vi "Historical Warnings (SubVI).vi"(7 "Warnings bool array":bool[](array[boolean]), 8 "in":bool, 11 "warnings table in":T1(array[cluster]) {"Time Stamp" format="%<%.3X %x>T"}) -> (3 "Warnings table out":T1(array[cluster]) {"Time Stamp" format="%<%.3X %x>T"})   [LabVIEW 2022 SP3]
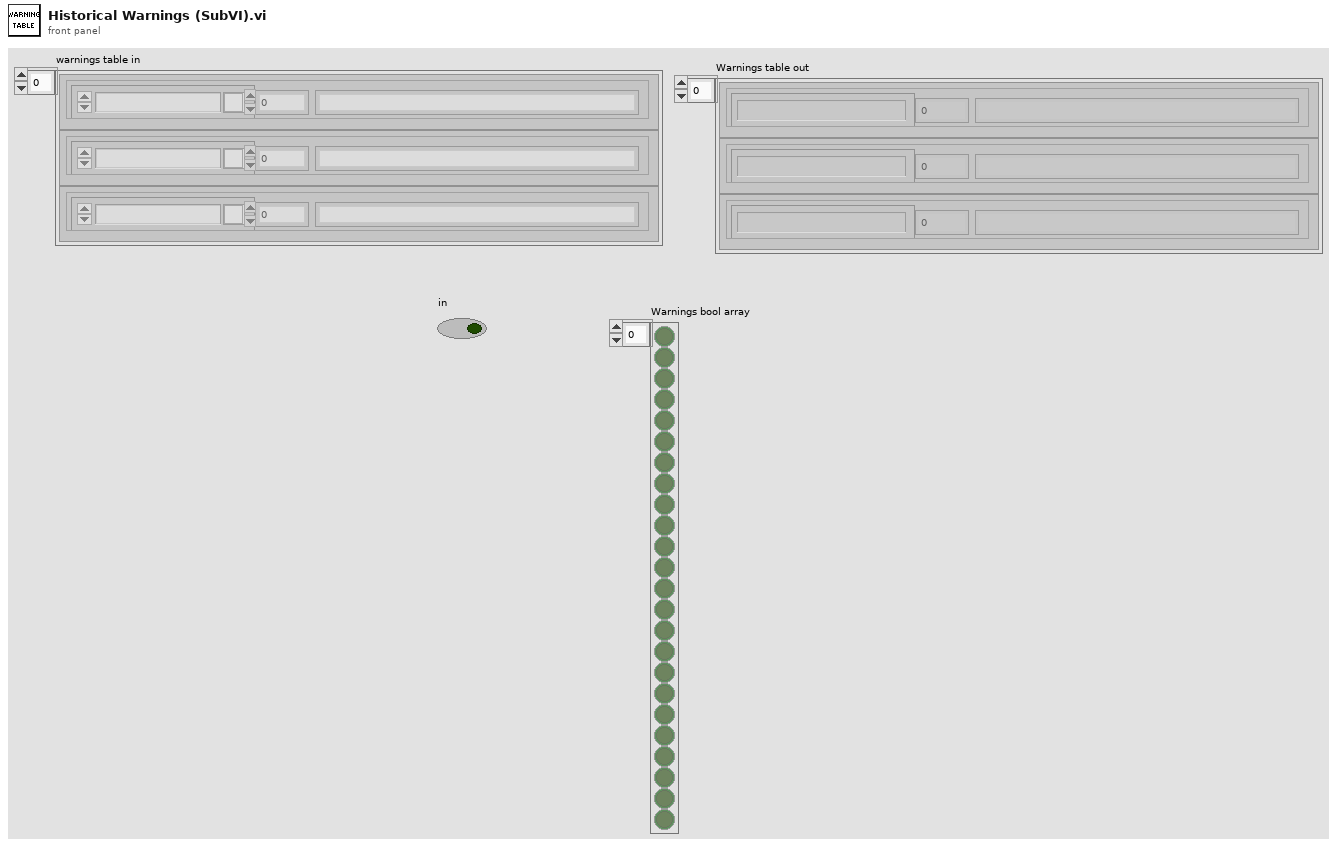
[diagram p1: front panel]
types:
  T1 = cluster{"Time Stamp":timestamp, "Descripcion":string, "Numeric":i32}[]
  T2 = cluster{"Time Stamp":timestamp, "Descripcion":string, "Numeric":i32}
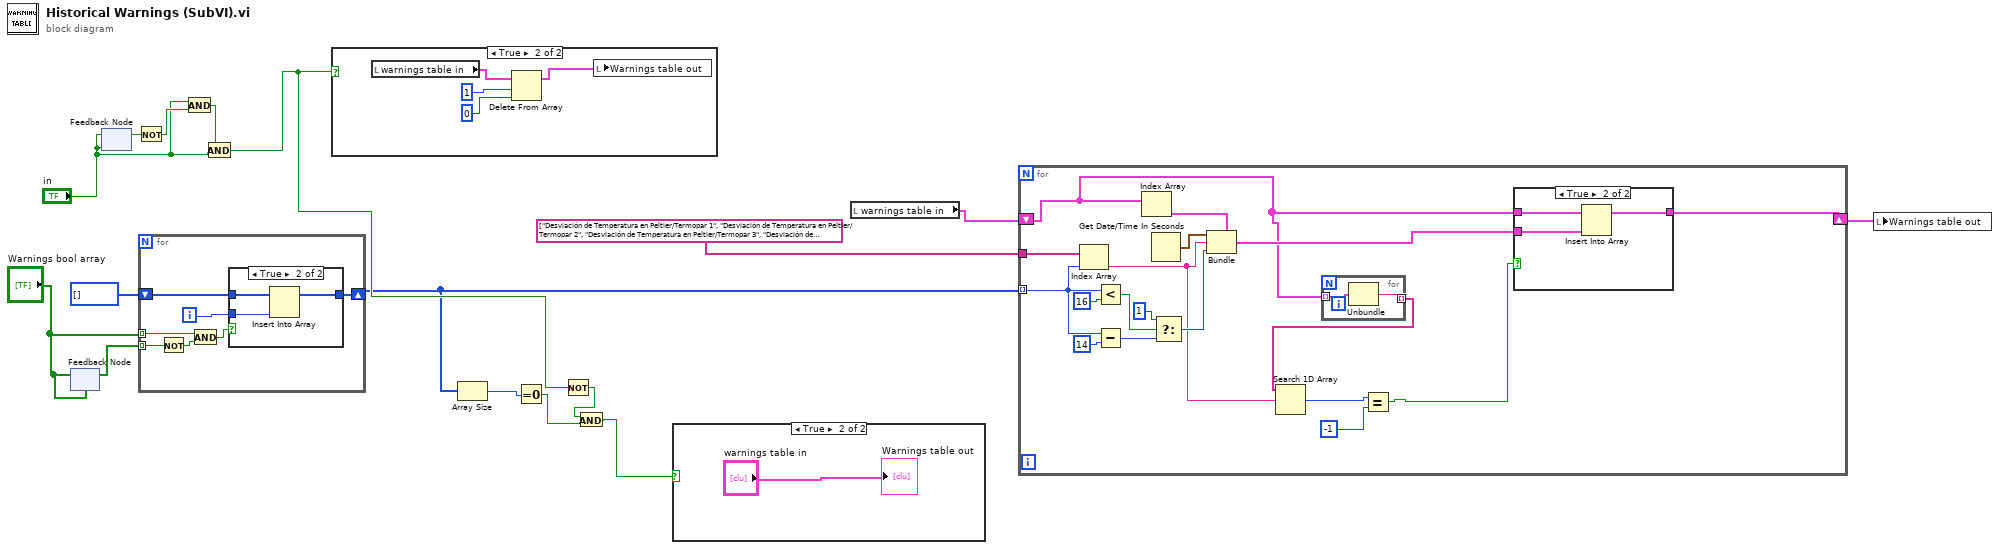
[diagram p0: block diagram]
diagram:
  n1 = feedback #1("Warnings bool array") -> (w13:bool[])
  n2 = feedback-in #1("Warnings bool array") -> ()
  n3 = feedback #2("in") -> (w10:bool)
  n4 = feedback-in #2("in") -> ()
  n5 = Not(x=w10) -> (.not. x?=w11:bool)
  n6 = for {
    tunnel: w13 -> [w23] mode=indexing
    tunnel: "Warnings bool array" -> [w21] mode=indexing
    shift-right: [w17] -> w3
    shift-left: i32[] [] -> [w20]
    i -> [w19]
    n7 = Not(x=w23) -> (.not. x?=w22:bool)
    n8 = And(x=w21, y=w22) -> (x .and. y?=w18:bool)
    n9 = case shown="True" w18 {
      tunnel: w20 -> [w24 w27]
      tunnel: w19 -> [_ w25]
      tunnel: [w24 w26] -> w17
      frame False {
      }
      frame True {
        n10 = Insert Into Array(array=w27, new element=w25) -> (w26:i32[])  [unwired: 1 in]
      }
    }
  }
  n11 = And(x="in", y=w11) -> (x .and. y?=w9:bool)
  n12 = And(x=w9, y="in") -> (x .and. y?=w5:bool)
  n13 = case shown="True" w5 {
    frame False {
    }
    frame True {
      n14 = local read "warnings table in"() -> (w30:T1)
      n15 = Delete From Array(array=w30, length=1, index=0) -> (array with subset deleted=w31:T1)  [unwired: 1 out]
      n16 = local write "Warnings table out"(w31) -> ()
    }
  }
  n17 = Array Size(array=w3) -> (size(s)=w12:i32)
  n18 = Equal To 0?(x=w12) -> (x = 0?=w7:bool)
  n19 = Not(x=w5) -> (.not. x?=w6:bool)
  n20 = And(x=w6, y=w7) -> (x .and. y?=w4:bool)
  n21 = case shown="True" w4 {
    frame False {
    }
    frame True {
      "Warnings table out" <- "warnings table in"
    }
  }
  n22 = local read "warnings table in"() -> (w2:T1)
  n23 = for {
    tunnel: w3 -> [w40] mode=indexing
    tunnel: string[] ["Desviación de Temperatura en Peltier/Termopar 1", "Desviación de Temperatura en Peltier/Termopar 2", "Desviación de Temperatura en Peltier/Termopar 3", "Desviación de Temperatura en Peltier/Termopar 4", "Desviación de Temperatura en Peltier/Termopar 5", "Desviación de Temperatura en Peltier/Termopar 6", "Desviación de Temperatura en Peltier/Termopar 7", "Desviación de Temperatura en Peltier/Termopar 8", "Desviación de Temperatura en Peltier/Termopar 9", "Desviación de Temperatura en Peltier/Termopar 10", "Desviación de Temperatura en Peltier/Termopar 11", "Desviación de Temperatura en Peltier/Termopar 12", "Desviación de Temperatura en Peltier/Termopar 13", "Desviación de Temperatura en Peltier/Termopar 14", "Desviación de Temperatura en Peltier/Termopar 15", "Desviación de Temperatura en Peltier/Termopar 16", "Desviación de Temperatura en la CC.", "Disparo del valor LEL (%). AMBIENTE EXPLOSIVO", "Valor anómalo de O2(%)"] -> [w47]
    shift-right: [w39] -> w1
    shift-left: w2 -> [w36]
    n24 = Index Array(array=w47, index=w40) -> (element=w37:string)
    n25 = Less?(x=w40, y=16) -> (x < y?=w45:bool)
    n26 = Subtract(x=w40, y=14) -> (x-y=w42:i32)
    n27 = Index Array(array=w36) -> (element=w49:T2)  [unwired: 1 in]
    n28 = Get Date/Time In Seconds() -> (seconds since 1Jan1904=w48:timestamp)
    n29 = Select(t=1, s=w45, f=w42) -> (s? t:f=w41:i32)
    n30 = Bundle(cluster=w49, "Time Stamp"=w48, "Descripcion"=w37, "Numeric"=w41) -> (w50:T2)
    n31 = for {
      tunnel: w36 -> [w56] mode=indexing
      tunnel: [w55] -> w38 mode=indexing
      n32 = Unbundle(w56) -> ("Descripcion"=w55:string)  [unwired: 2 out]
    }
    n33 = Search 1D Array(1D array=w38, element=w37) -> (index of element=w35:i32)  [unwired: 1 in]
    n34 = Equal?(x=w35, y=-1) -> (x = y?=w34:bool)
    n35 = case shown="True" w34 {
      tunnel: w50 -> [_ w54]
      tunnel: [w51 w53] -> w39
      tunnel: w36 -> [w51 w52]
      frame False {
      }
      frame True {
        n36 = Insert Into Array(array=w52, new element=w54) -> (w53:T1)  [unwired: 1 in]
      }
    }
  }
  n37 = local write "Warnings table out"(w1) -> ()
